vi "Dashboard Main.vi"() -> ()   [LabVIEW 2016]
uses:
  <vilib>/vision/Image Controls.llb/IMAQ Image.ctl
  <vilib>/Utility/miscctls.llb/LVRowAndColumnTypeDef.ctl
  <vilib>/event_ctls.llb/eventvkey.ctl
  <vilib>/Rock Robotics/Network Tables/NT Read Boolean.vi
  <vilib>/Rock Robotics/Network Tables/NT Read Numeric Array.vi
  <vilib>/Rock Robotics/Network Tables/NT Read Boolean Array.vi
  <vilib>/Rock Robotics/WPI/Dashboard/WPI_DashboardLogging Global.vi
  <vilib>/vision/NI_Vision_Development_Module.lvlib
panel:
  in  "Camera Settings Right":T1={"Frame Rate"=30, "Compression"=30, "Size"=1, "DB Camera Config"=FALSE} {"Frame Rate" scale=1.0..30.0; "Compression" scale=100.0..-1.0; "Size" items=["640x480", "320x240", "160x120"]}
  in  "Camera2 Name":string(combo)="Camera2"
  out "Camera Info":cluster{"Mbps LED":bool, "Mbps":dbl, "fps":dbl} {"fps" format="%#.1g"; "Mbps" format="%#.1g"}
  in  "Camera Settings":T1={"Frame Rate"=30, "Compression"=30, "Size"=1, "DB Camera Config"=FALSE} {"Frame Rate" scale=1.0..30.0; "Compression" scale=100.0..-1.0; "Size" items=["640x480", "320x240", "160x120"]}
  in  "TCP":refnum<k5>
  in  "Rec Mode":enum32{"Stop", "Record", "Playback"}(radio)
  out "Robot IP":string
  out "Image Message":string="Timeout in Camera Communications"
  in  "Dashboard Tab":T2(tab)
  in  "Ball Picker Upper Speed":dbl=1.0
  out "Shooter RPM":dbl
  in  "Select Auto":string(combo)="Select Autonomous ..."
  out "NT Connection":bool
  out "MotorChart R":cluster{"Numeric":dbl, "Numeric":dbl}(graph)
  out "MotorChart L":cluster{"Numeric":dbl, "Numeric":dbl}(graph)
  out "MotorSliders R":cluster{"MotorSlide1":dbl, "MotorSlide2":dbl} {"MotorSlide2" scale=-1.0..1.0 scale format="%#_2e"; "MotorSlide1" scale=-1.0..1.0 scale format="%#_2e"}
  out "MotorSliders L":cluster{"MotorSlide1":dbl, "MotorSlide2":dbl} {"MotorSlide2" scale=-1.0..1.0 scale format="%#_2e"; "MotorSlide1" scale=-1.0..1.0 scale format="%#_2e"}
  out "JS1 Z":dbl(slide) scale=-1.0..1.0 scale format="%#_2e"
  out "JS1 Graph":cluster{"X":dbl, "Y":dbl}[](graph)
  out "JS1 Buttons":T3
  out "JS2 Z":dbl(slide) scale=-1.0..1.0 scale format="%#_2e"
  out "JS2 Graph":cluster{"X":dbl, "Y":dbl}[](graph)
  out "JS2 Buttons":T3
  out "Mode":T4(ring)=enum."Auto Disabled"
  out "Drive Direction":enum32{"Gear/Climb", "Ball Picking/Shooting"}(tab)
  out "Gear Holder Position":T5(tab)
  out "Climber Speed":dbl format="%#_2g"
  out "Tab Control":enum32{"Dont Shoot", "SHOOT"}(tab)
  out "Shooter RPM":dbl
  out "Gear Holder Position 2":T6(tab)
  out "LIDAR":dbl
  in  "Drive Forward Auto Wait":dbl
  in  "Distance for 5500RPM":dbl=7.0 format="%#_13g"
  out "Ball Motor Direction":bool
  out "Camera Image Right":T7(plugin-control)
  in  "DB/String 9":string
  in  "DB/String 8":string
  in  "DB/String 7":string
  in  "DB/String 6":string
  in  "DB/String 5":string
  in  "DB/String 4":string
  in  "DB/String 3":string
  in  "DB/String 2":string
  in  "DB/String 1":string
  in  "DB/String 0":string
  in  "DB/Slider 0":dbl(slide) scale=0.0..5.0
  in  "DB/Slider 1":dbl(slide) scale=0.0..5.0
  in  "DB/Slider 2":dbl(slide) scale=0.0..5.0
  in  "DB/Slider 3":dbl(slide) scale=0.0..5.0
  out "DB/LED 3":bool
  out "DB/LED 2":bool
  out "DB/LED 1":bool
  out "DB/LED 0":bool
  in  "DB/Button 3":bool
  in  "DB/Button 2":bool
  in  "DB/Button 1":bool
  in  "DB/Button 0":bool caption="New Name"
  out "Teleop Variables":string[][](array[string])
  in  "Test Slider":dbl(slide) scale=0.0..100.0 scale format="%#_3g"
  in  "On/Off":bool caption="Solenoid"
  in  "Test Name":u16(ring) items=["Select the test to run..."]
  in  "Test Tree":string(tree)
  in  "Motor":cluster{"Value":dbl, "Enable":bool} {"Value" scale=-1.0..1.0 scale format="%#_3g"}
  out "Progress":T8 {"Test Progress" scale=0.0..100.0}
  in  "Rev/Fwd":cluster{"Forward":bool, "Reverse":bool}
  in  "Test Ring":u16(ring) items=["Monochrome", "Color"]
  out "Cmd Status":string
  in  "Execute Command":bool
  in  "Command Params":string[][](table)
  in  "Command Selection":i32(listbox)
  in  "CheckList":i32(listbox)
  out "Tree":string(tree)
  out "Camera Image":T7(plugin-control)
  out "Background":bool
  in  "Camera Name":string(combo)="Camera"
  # "HW"
  # "HW"
  # "Joysticks"
  # "Drive Motors"
  # "Front"
  # "Right"
  # "Left"
  # "Back"
  # "Gear and Climber"
  # "NEITHER SWITCH PRESSED"
  # "Ball Picking/Shooting"
  # "DONT SHOOT"
  # "SHOOT"
  # "This tab is a great place for autonomous settings and robot-specific values.\nPlace controls and indicators inside this tab and match name to\nDashboard Variables on robot. You can also delete this comment."
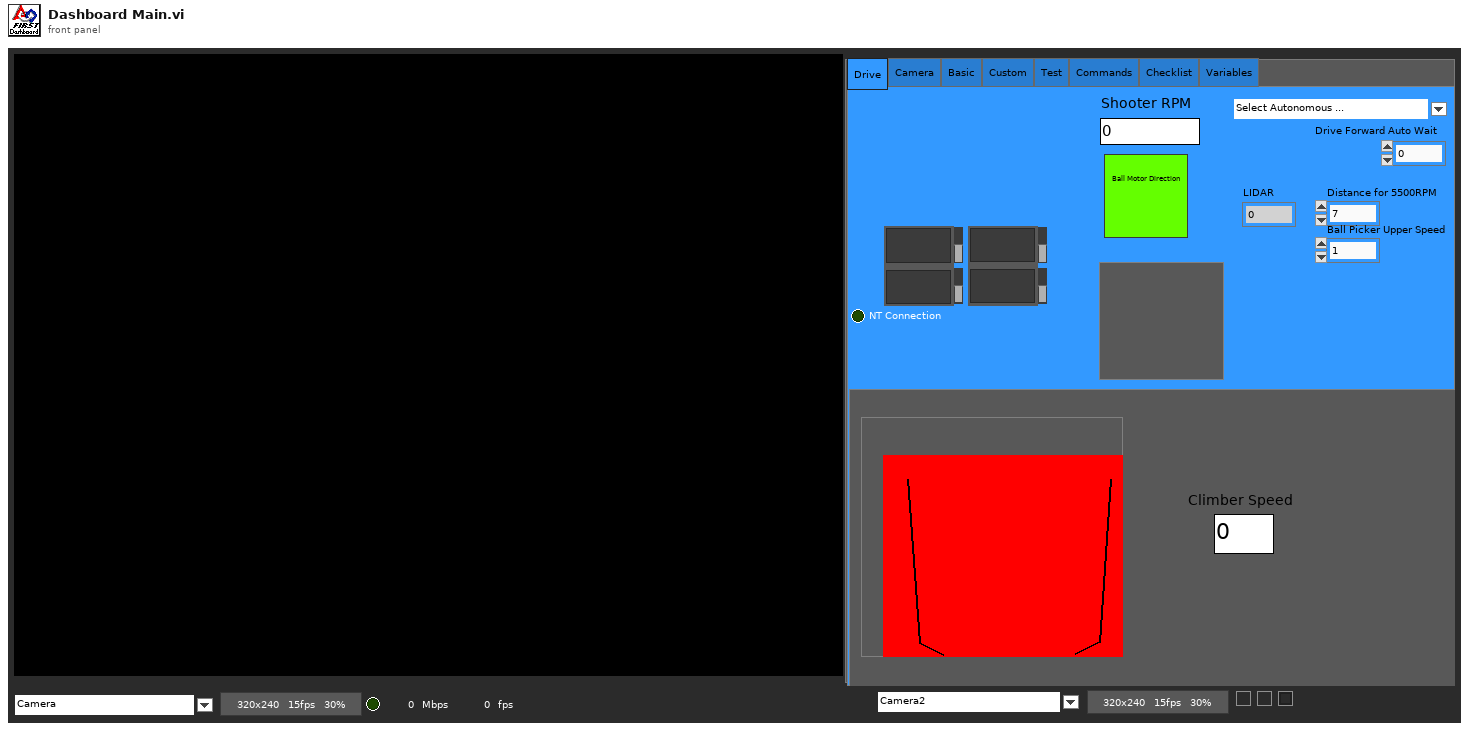
[diagram p1: front panel]
types:
  T1 = cluster{"Frame Rate":i32, "Compression":i32, "Size":u16, "DB Camera Config":bool}
  T2 = enum32{"Drive", "Camera", "Basic", "Custom", "Test", "Commands", "Checklist", "Variables"}
  T3 = cluster{bool, bool, bool, bool, bool, bool, bool, bool, bool, bool, bool, bool}
  T4 = enum8{"Tele-Op Disabled", "Tele-Op Enabled", "Auto Disabled", "Auto Enabled", "Test Disabled", "Test Enabled", "Disconnected", "No Code", "E-Stop"}
  T5 = enum32{"Gear Release Position", "Gear Hold Position", "NA"}
  T6 = enum32{"Gear Release Position", "Gear Hold Position"}
  T7 = typedef "IMAQ Image.ctl" = refnum<image>
  T8 = cluster{"Test Progress":u8, "Test Progress Text":string}
  T9 = typedef "Image Type" = u32
  T10 = cluster{"IDs":cluster{"RPC field ID":u16, "Unique ID":u16}, "String":string}
  T11 = enum32{"Drive", "Basic", "Custom", "Test", "Checklist", "Variables"}
  T12 = cluster{"Camera Image":refnum<vi>, "Dashboard Tab":refnum<vi>, "Background":refnum<vi>, "Rec Mode":refnum<vi>, "Test Slider":refnum<vi>, "On/Off ":refnum<vi>, "Test Ring":refnum<vi>, "Rev/Fwd":refnum<vi>, "Test Name":refnum<vi>, "Motor":refnum<vi>, "Progress":refnum<vi>, "CheckList":refnum<vi>, "Tree":refnum<vi>, "Test Tree":refnum<vi>, "Command Params":refnum<vi>, "Command Selection":refnum<vi>, "Execute Command":refnum<vi>, "Cmd Status":refnum<vi>, "Camera Settings":refnum<vi>, "Camera Name":refnum<vi>, "Camera Info":refnum<vi>, "Camera Settings Right":refnum<vi>, "Camera2 Name":refnum<vi>, "Camera Image Right":refnum<vi>}
  T13 = cluster{"Error Strings":string, "Disable Counts":cluster{u16, u16}, "Rail Faults":cluster{u16, u16, u16}, "Robot IP":string, "DB Mode":u8, "Event Info":cluster{"Name":string, "Type":u8, "Number":u16, "Replay":u8}}
  T14 = cluster{"Storage":cluster{"Disk Free":u64, "RAM Block":u32, "RAM free":u32}, "CPU Utilization":cluster{"CPU % ISR":sgl, "CPU % Time Crit":sgl, "CPU % Timed Str":sgl, "CPU % High":sgl, "CPU % Above":sgl, "CPU % Normal":sgl, "CPU % Low":sgl}, "CAN":cluster{"% Bus Utilization":sgl, "Bus Off Cnt":u32, "TX_FIFO Full Cnt":u32, "Receive Error Cnt":u8, "Transmit Error Cnt":u8}, "HID":cluster{"HID Outputs":u32, "Rumble Low":u16, "Rumble High":u16}[]}
  T15 = cluster{"Status bits":cluster{"Test Mode":bool, "Autonomous":bool, "Enabled":bool, "Code Start":bool, "Brownout":bool, "Reserved 2":bool, "Reserved 3":bool, "E-Stop":bool}, "Code Trace":cluster{"Disabled":bool, "TeleOp":bool, "Auto":bool, "Test":bool}, "Controller Type":enum16{"unknown", "cRIO", "roboRio"}, "Code?":enum16{"unknown", "noCode", "code"}, "Battery V":dbl}
  T16 = cluster{"Control Bits":cluster{"TestMode":bool, "Autonomous":bool, "Enabled":bool, "FMS Present":bool, bool, bool, bool, "E-Stop":bool}, "Team Station ":u8, "Countdown":sgl, "Joystick Values":cluster{"Axes":dbl[], "Buttons":bool[], "POVs":i16[]}[]}
  T17 = cluster{"Axes":dbl[], "Buttons":bool[], "POVs":i16[]}[]
  T18 = cluster{"Axes":dbl[], "Buttons":bool[], "POVs":i16[]}
  T19 = cluster{"Buttons[0]":bool, "Buttons[1]":bool, "Buttons[2]":bool, "Buttons[3]":bool, "Buttons[4]":bool, "Buttons[5]":bool, "Buttons[6]":bool, "Buttons[7]":bool, "Buttons[8]":bool, "Buttons[9]":bool, "Buttons[10]":bool, "Buttons[11]":bool}
  T20 = cluster{"Operation":enum16{"Update", "Clear"}, "Color Box":u32}[]
  T21 = typedef "eventvkey.ctl" = enum16{"ASCII", "Enter", "Return", "Shift", "Ctrl", "Alt", "Cmd", "Opt", "Caps", "NumLock", "Clear", "Break", "Up", "Down", "Left", "Right", "Insert", "Delete", "Home", "End", "PageUp", "PageDown", "Escape", "Help", "Pause", "ScrollLock", "F1", "F2", "F3", "F4", "F5", "F6", "F7", "F8", "F9", "F10", "F11", "F12", "F13", "F14", "F15", "F16", "F17", "F18", "F19", "F20", "F21", "F22", "F23", "F24", "Play", "VolumeUp", "VolumeDown", "Mute", "Two Byte Char"}
  T22 = cluster{"Image Size":bool, "Image Type":bool, "Pixel Value":bool, "ROI Information":bool, "Zoom Factor":bool}
  T23 = cluster{"Operation":enum16{"Update", "Clear"}, "Color Box":u32}
  T24 = typedef "LVRowAndColumnTypeDef.ctl" = cluster{"Row":i32, "Column":i32}
  T25 = cluster{"Shift":bool, "Ctrl":bool, "Alt":bool, "Cmd":bool, "Opt":bool}
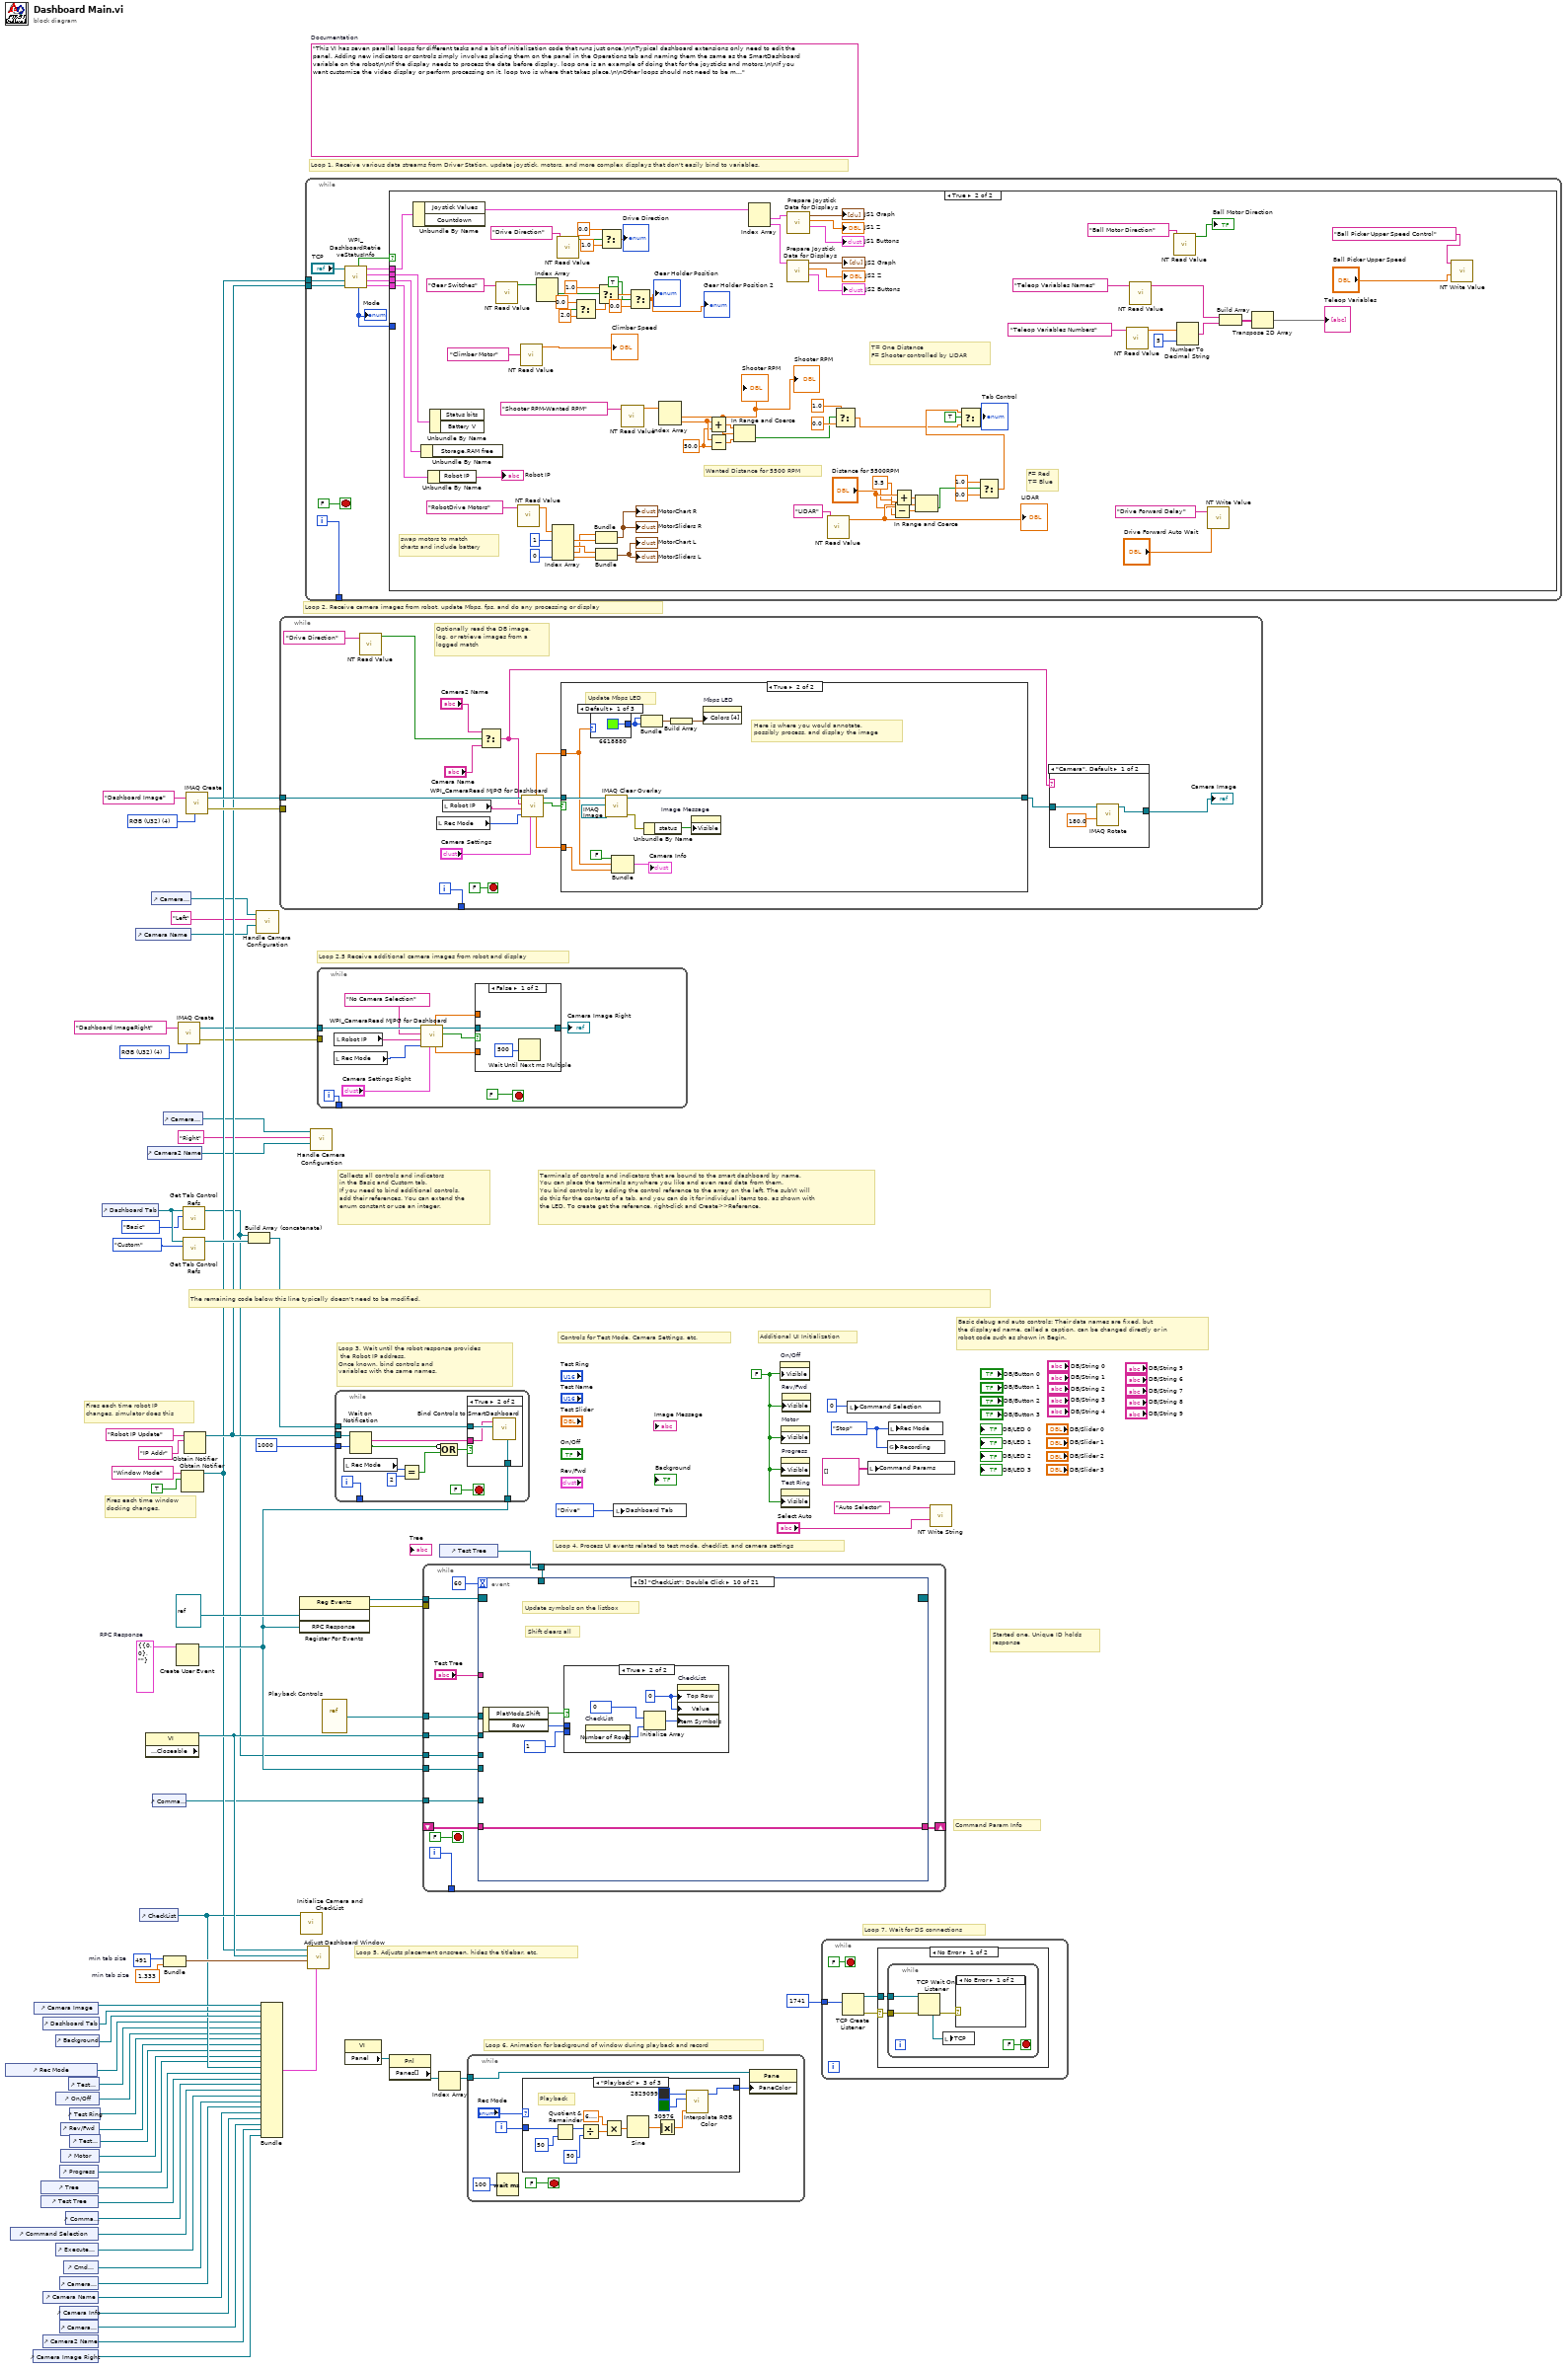
[diagram p0: block diagram]
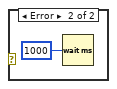
[diagram p3: hidden frame]
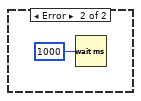
[diagram p4: hidden frame]
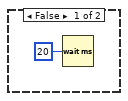
[diagram p5: hidden frame]
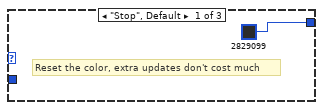
[diagram p6: hidden frame]
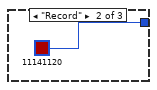
[diagram p7: hidden frame]
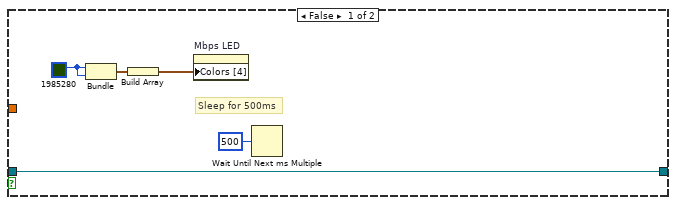
[diagram p10: hidden frame]
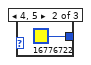
[diagram p11: hidden frame]
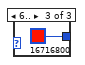
[diagram p12: hidden frame]
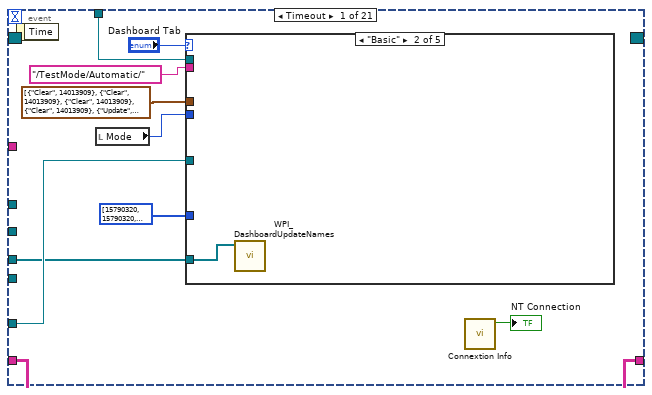
[diagram p13: hidden frame]
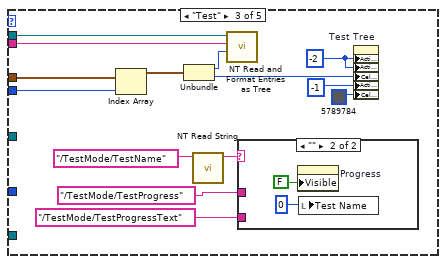
[diagram p15: hidden frame]
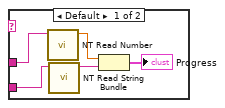
[diagram p16: hidden frame]
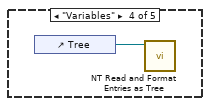
[diagram p17: hidden frame]
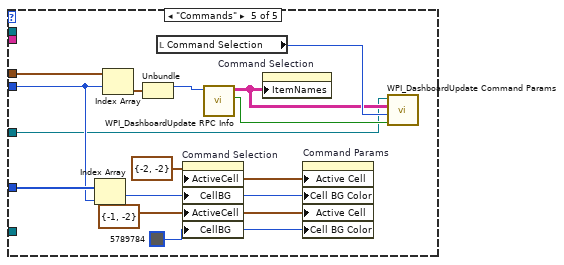
[diagram p18: hidden frame]
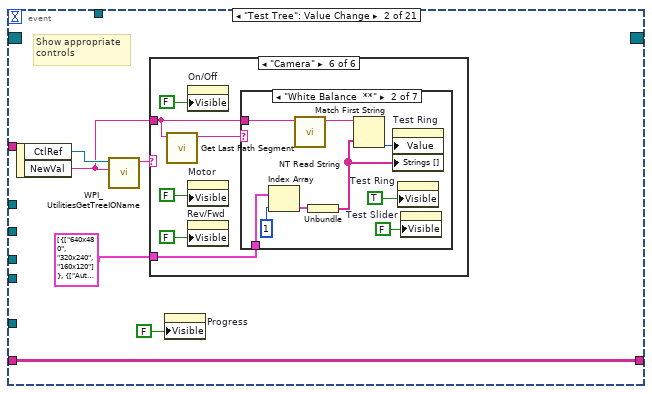
[diagram p19: hidden frame]
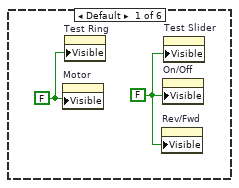
[diagram p20: hidden frame]
diagram:
  (unwired) T7 refnum ("Camera Image")
  w10 = T9 4 items=["Grayscale (U8)", "Grayscale (I16)", "Grayscale (SGL)", "Complex (CSG)", "RGB (U32)", "HSL (U32)", "RGB (U64)"] ("Image Type")
  w26 = T10 {"IDs"={"RPC field ID"=0, "Unique ID"=0}, "String"=""}  # RPC Response
  w51 = 491  # min tab size
  w50 = 1.333  # min tab size
  w58 = enum32{"Stop", "Record", "Playback"}."Stop" ("Rec Mode")
  w33 = FALSE ("Visible")
  (unwired) "This VI has seven parallel loops for different tasks and a bit of initialization code that runs just once.\n\nTypical dashboard extensions only need to edit the panel. Adding new indicators or controls simply involves placing them on the panel in the Operations tab and naming them the same as the SmartDashboard variable on the robot\n\nIf the display needs to process the data before display, loop one is an example of doing that for the joysticks and motors.\n\nIf you want customize the video display or perform processing on it, loop two is where that takes place.\n\nOther loops should not need to be modified. They are pretty standard, and document the task they perform."  # Documentation
  w75 = T9 4 items=["Grayscale (U8)", "Grayscale (I16)", "Grayscale (SGL)", "Complex (CSG)", "RGB (U32)", "HSL (U32)", "RGB (U64)"] ("Image Type")
  # "Loop 2.5 Receive additional camera images from robot and display"
  # "Command Param Info"
  # "Started one, Unique ID holds\nresponse"
  # "Loop 7. Wait for DS connections"
  # "Basic debug and auto controls: Their data names are fixed, but\nthe displayed name, called a caption, can be changed directly or in\nrobot code such as shown in Begin."
  # "Controls for Test Mode, Camera Settings, etc."
  # "Additional UI Initialization"
  # "Loop 6. Animation for background of window during playback and record"
  # "Fires each time robot IP\nchanges, simulator does this"
  # "Fires each time window\ndocking changes."
  # "Collects all controls and indicators\nin the Basic and Custom tab.\nIf you need to bind additional controls,\nadd their references. You can extend the\nenum constant or use an integer."
  # "The remaining code below this line typically doesn't need to be modified."
  # "Loop 4. Process UI events related to test mode, checklist, and camera settings"
  # "Terminals of controls and indicators that are bound to the smart dashboard by name.\nYou can place the terminals anywhere you like and even read data from them.\nYou bind controls by adding the control reference to the array on the left. The subVI will\ndo this for the contents of a tab, and you can do it for individual items too, as shown with\nthe LED. To create get the reference, right-click and Create>>Reference."
  # "Loop 3. Wait until the robot response provides\n the Robot IP address.\nOnce known, bind controls and\nvariables with the same names."
  # "Loop 5. Adjusts placement onscreen, hides the titlebar, etc."
  # "Loop 1. Receive various data streams from Driver Station, update joystick, motors, and more complex displays that don't easily bind to variables."
  # "Loop 2. Receive camera images from robot, update Mbps, fps, and do any processing or display"
  n1 = control-ref of="Rec Mode"() -> (w39:refnum<vi>)
  n2 = control-ref of="Command Selection"() -> (w25:refnum<vi>)
  n3 = control-ref of="Camera Image Right"() -> (w1:refnum<vi>)
  n4 = control-ref of="Camera Image"() -> (w53:refnum<vi>)
  n5 = control-ref of="Tree"() -> (w43:refnum<vi>)
  n6 = control-ref of="Test Tree"() -> (w42:refnum<vi>)
  n7 = control-ref of="Dashboard Tab"() -> (w52:refnum<vi>)
  n8 = control-ref of="Camera Name"() -> (w16:refnum<vi>)
  n9 = control-ref of="Camera2 Name"() -> (w2:refnum<vi>)
  n10 = control-ref of="Execute Command"() -> (w27:refnum<vi>)
  n11 = control-ref of="Background"() -> (w48:refnum<vi>)
  n12 = control-ref of="On/Off"() -> (w37:refnum<vi>)
  n13 = control-ref of="Progress"() -> (w34:refnum<vi>)
  n14 = control-ref of="Camera Settings"() -> (w17:refnum<vi>)
  n15 = control-ref of="Camera Info"() -> (w15:refnum<vi>)
  n16 = control-ref of="Camera Settings Right"() -> (w3:refnum<vi>)
  n17 = control-ref of="Rev/Fwd"() -> (w35:refnum<vi>)
  n18 = control-ref of="Motor"() -> (w40:refnum<vi>)
  n19 = control-ref of="Cmd Status"() -> (w21:refnum<vi>)
  n20 = control-ref of="Command Params"() -> (w28:refnum<vi>)
  n21 = control-ref of="Test Slider"() -> (w38:refnum<vi>)
  n22 = control-ref of="Test Ring"() -> (w36:refnum<vi>)
  n23 = control-ref of="Test Name"() -> (w41:refnum<vi>)
  n24 = control-ref of="Dashboard Tab"() -> (w56:refnum<vi>)
  n25 = control-ref of="Camera Name"() -> (w18:refnum<vi>)
  n26 = control-ref of="CheckList"() -> (w44:refnum<vi>)
  n27 = property class="VI" props=["Front Panel.Closeable"]() -> (reference out=w57:refnum<vi>)  [unwired: 2 in, 2 out]
  n28 = control-ref of="Camera2 Name"() -> (w6:refnum<vi>)
  n29 = control-ref of="Camera Settings"() -> (w19:refnum<vi>)
  n30 = control-ref of="Command Params"() -> (w20:refnum<vi>)
  n31 = control-ref of="Camera Settings Right"() -> (w7:refnum<vi>)
  n32 = Bundle("min tab size"=w51, "min tab size"=w50) -> (w49:cluster{"min tab size":i32, "min tab size":dbl})  [unwired: 1 in]
  n33 = Create User Event(user event datatype=w26) -> (user event=w22:refnum<user-event>)  [unwired: 1 in, 1 out]
  n34 = call "IMAQ Create"("Image Name"="Dashboard ImageRight", "Image Type"=w10) -> ("New Image"=w9:T7, "error out"=w8:errorcluster)  [unwired: 2 in, 1 out]
  n35 = Obtain Notifier(name (unnamed)="Window Mode", notification data type=TRUE) -> (notifier out=w31:refnum<notifier>)  [unwired: 2 in, 2 out]
  n36 = call <vilib>:"Get Tab Control Refs.vi"("Page Index"=T11."Basic" ("Dashboard Tab"), "TabControl in"=w56) -> ("ControlsOnPage"=w14:refnum<vi>[])  [unwired: 9 in]
  n37 = call <vilib>:"Get Tab Control Refs.vi"("Page Index"=T11."Custom" ("Dashboard Tab"), "TabControl in"=w56) -> ("ControlsOnPage"=w55:refnum<vi>[])  [unwired: 9 in]
  n38 = Obtain Notifier(name (unnamed)="Robot IP Update", notification data type="IP Addr" ("name (unnamed)")) -> (notifier out=w32:refnum<notifier>)  [unwired: 2 in, 2 out]
  n39 = call "IMAQ Create"("Image Name"="Dashboard Image", "Image Type"=w75) -> ("New Image"=w73:T7, "error out"=w72:errorcluster)  [unwired: 2 in, 1 out]
  n40 = Build Array (concatenate)(w14, w55) -> (w54:refnum<vi>[])
  n41 = call "Handle Camera Configuration.vi"("CameraNameRef"=w18, "Camera File Name"="Left", "ClusterRef"=w19) -> ()  [unwired: 9 in]
  n42 = Bundle("Camera Image"=w53, "Dashboard Tab"=w52, "Background"=w48, "Rec Mode"=w39, "Test Slider"=w38, "On/Off"=w37, "Test Ring"=w36, "Rev/Fwd"=w35, "Test Name"=w41, "Motor"=w40, "Progress"=w34, "CheckList"=w44, "Tree"=w43, "Test Tree"=w42, "Command Params"=w28, "Command Selection"=w25, "Execute Command"=w27, "Cmd Status"=w21, "Camera Settings"=w17, "Camera Name"=w16, "Camera Info"=w15, "Camera Settings Right"=w3, "Camera2 Name"=w2, "Camera Image Right"=w1) -> (w45:T12)  [unwired: 1 in]
  n43 = while {
    tunnel: w73 -> [w90]
    tunnel: w72 -> [_]
    tunnel: [w91] -> _
    i -> [w91]
    stop <- FALSE stop-if-true
    # "Optionally read the DB image,\nlog, or retrieve images from a\nlogged match"
    n44 = call-poly <vilib>:"NT Read Value.vi"("Name"="Drive Direction") -> ("Boolean"=w77:bool)  [unwired: 9 in, 1 out]
    n45 = local read "Rec Mode"() -> (w86:enum32{"Stop", "Record", "Playback"})
    n46 = local read "Robot IP"() -> (w85:string)
    n47 = Select(t="Camera2 Name", s=w77, f="Camera Name") -> (s? t:f=w76:string)
    n48 = call <vilib>:"WPI_CameraRead MJPG for Dashboard.vi"("Camera Settings"="Camera Settings", "Rec Mode"=w86, "Robot IP"=w85, "Camera Name"=w76, "Refnum in"=w90) -> ("Active"=w88:bool, "Refnum out"=w89:T7, "FPS"=w87:dbl, "Bandwidth (Mbps)"=w84:dbl)  [unwired: 3 in]
    n49 = case shown="True" w88 {
      tunnel: w89 -> [w97 w108]
      tunnel: w84 -> [_ w105]
      tunnel: w87 -> [_ w106]
      tunnel: [w97 w102] -> w78
      frame False {
        w99 = u32 1985280 ("Color Box")
        # "Sleep for 500ms"
        n50 = Bundle("Color Box"=w99, "Color Box"=w99) -> (w100:cluster{"Color Box":u32, "Color Box":u32})  [unwired: 1 out]
        n51 = Build Array(w100) -> (w98:cluster{"Color Box":u32, "Color Box":u32}[])
        n52 = property on="Mbps LED" class="Bool (strict)"("Colors [4]"=w98) -> ()  [unwired: 2 in, 2 out]
        n53 = Wait Until Next ms Multiple(millisecond multiple=u32 500) -> ()  [unwired: 1 out]
      }
      frame True {
        # "Here is where you would annotate,\npossibly process, and display the image"
        # "Update Mbps LED"
        n54 = case shown="Default" w105 {
          tunnel: [u32 6618880 ("Color Box") u32 16776722 ("Color Box") u32 16716800 ("Color Box")] -> w109
          frame Default {
          }
          frame 4, 5 {
          }
          frame 6.. {
          }
        }
        n55 = call "IMAQ Clear Overlay"("Image"=w108) -> ("error out"=w111:errorcluster, "Image Out"=w102:T7)  [unwired: 2 in, 7 out]
        n56 = Bundle(FALSE, "Bandwidth (Mbps)"=w105, "FPS"=w106) -> (→"Camera Info":cluster{bool, "Bandwidth (Mbps)":dbl, "FPS":dbl})  [unwired: 1 in]
        n57 = Bundle("Color Box"=w109, "Color Box"=w109) -> (w110:cluster{"Color Box":u32, "Color Box":u32})  [unwired: 1 out]
        n58 = Unbundle By Name(w111) -> ("status"=w112:bool)
        n59 = Build Array(w110) -> (w107:cluster{"Color Box":u32, "Color Box":u32}[])
        n60 = property on="Image Message" class="Str"("Visible"=w112) -> ()  [unwired: 2 in, 2 out]
        n61 = property on="Mbps LED" class="Bool (strict)"("Colors [4]"=w107) -> ()  [unwired: 2 in, 2 out]
      }
    }
    n62 = case shown="\"Camera\", Default" w76 {
      tunnel: [w94 w96] -> w79
      tunnel: w78 -> [w95 w96]
      frame "Camera", Default {
        n63 = call "IMAQ Rotate"("Angle (degrees)"=sgl 180.0, "Image Src"=w95) -> ("Image Dst Out"=w94:T7)  [unwired: 8 in, 1 out]
      }
      frame "Camera2" {
      }
    }
    "Camera Image" <- w79
  }
  n64 = register-events(refnum<vi> refnum, w22) -> (reference out=w62:refnum<event-registration>, error out=w61:errorcluster)  [unwired: 2 in]
  n65 = call "Initialize Camera and CheckList.vi"("ListBox in"=w44) -> ()  [unwired: 11 in]
  n66 = while {
    tunnel: [w125] -> _
    tunnel: w32 -> [w119]
    tunnel: w31 -> [w116]
    i -> [w125]
    stop <- FALSE stop-if-true
    n67 = call <vilib>:"WPI_DashboardRetrieveStatusInfo.vi"("Binding Refnum"=w119, "Window Mode Notifier"=w116, "TCP Cnx"="TCP") -> ("Power and Errors"=w120:T13, "Robot Metrics"=w123:T14, "Status Info"=w124:T15, "Control Info"=w121:T16, "Robot Mode"=w118:T4, "Process?"=w122:bool)  [unwired: 3 in]
    "Mode" <- w118
    n68 = case shown="True" w122 {
      tunnel: w124 -> [_ w207]
      tunnel: w123 -> [_ w206]
      tunnel: w121 -> [_ w205]
      tunnel: w120 -> [_ w204]
      tunnel: w118 -> [_ _]
      frame False {
        n69 = Wait (ms)(milliseconds to wait=u32 20) -> ()  [unwired: 1 out]
      }
      frame True {
        w133 = 3.5 ("y")
        w149 = 50.0 ("y")
        # "T= One Distance\nF= Shooter controlled by LIDAR"
        # "Wanted Distance for 5500 RPM"
        # "F= Red\nT= Blue"
        # "swap motors to match\ncharts and include battery"
        n70 = Unbundle By Name(w205) -> ("Joystick Values"=w195:T17)  [unwired: 1 out]
        n71 = Unbundle By Name(w206) -> ()  [unwired: 1 out]
        n72 = Unbundle By Name(w204) -> ("Robot IP"=→"Robot IP":string)
        n73 = Unbundle By Name(w207) -> ()  [unwired: 2 out]
        n74 = call-poly <vilib>:"NT Read Value.vi"("Name"="Gear Switches") -> ("Boolean Array"=w167:bool[])  [unwired: 9 in, 1 out]
        n75 = call-poly <vilib>:"NT Read Value.vi"("Name"="RobotDrive Motors") -> ("Numeric Array"=w185:dbl[])  [unwired: 9 in, 1 out]
        n76 = call-poly <vilib>:"NT Read Value.vi"("Name"="Climber Motor") -> ("Numeric"=→"Climber Speed":dbl)  [unwired: 9 in, 1 out]
        n77 = Index Array(array=w167) -> (element #1=w166:bool, element #2=w164:bool)  [unwired: 2 in]
        n78 = Index Array(array=w185, index #1=1, index #4=0) -> (element #1=w199:dbl, element #2=w200:dbl, element #3=w198:dbl, element #4=w203:dbl)  [unwired: 2 in]
        n79 = call-poly <vilib>:"NT Read Value.vi"("Name"="Drive Direction") -> ("Boolean"=w172:bool)  [unwired: 9 in, 1 out]
        n80 = Select(t=0.0, s=w164, f=2.0) -> (s? t:f=w163:dbl)
        n81 = Bundle("Numeric"=w198, "Numeric"=w199) -> (→"MotorChart R" →"MotorSliders R":cluster{"Numeric":dbl, "Numeric":dbl})  [unwired: 1 in]
        n82 = Bundle("Numeric"=w200, "Numeric"=w203) -> (→"MotorChart L" →"MotorSliders L":cluster{"Numeric":dbl, "Numeric":dbl})  [unwired: 1 in]
        n83 = Select(t=1.0, s=w166, f=w163) -> (s? t:f=w158:dbl)
        n84 = Select(t=0.0, s=w172, f=1.0) -> (s? t:f=→"Drive Direction":dbl)
        n85 = call-poly <vilib>:"NT Read Value.vi"("Name"="Shooter RPM-Wanted RPM") -> ("Numeric Array"=w155:dbl[])  [unwired: 9 in, 1 out]
        n86 = Select(t=w158, s=TRUE, f=0.0) -> (s? t:f=→"Gear Holder Position" →"Gear Holder Position 2":dbl)
        n87 = Index Array(array=w155) -> (element #1=w147:dbl, element #2=w150:dbl)  [unwired: 2 in]
        "Shooter RPM" <- w147
        "Shooter RPM" <- w147
        n88 = Add(x=w150, y=w149) -> (x+y=w152:dbl)
        n89 = Subtract(x=w150, y=w149) -> (x-y=w151:dbl)
        n90 = In Range and Coerce(upper limit=w152, x=w147, lower limit=w151) -> (In Range?=w148:bool)  [unwired: 1 out]
        n91 = Index Array(array=w195) -> (element #1=w194:T18, element #2=w190:T18)  [unwired: 2 in]
        n92 = call "Prepare Joystick Data for Displays.vi"("Joystick Values"=w190) -> ("Buttons"=→"JS2 Buttons":T19, "Z Axis"=→"JS2 Z":dbl, "Cartesian Data"=→"JS2 Graph":cluster{"X axis":dbl, "X axis":dbl}[])  [unwired: 8 in]
        n93 = call "Prepare Joystick Data for Displays.vi"("Joystick Values"=w194) -> ("Buttons"=→"JS1 Buttons":T19, "Z Axis"=→"JS1 Z":dbl, "Cartesian Data"=→"JS1 Graph":cluster{"X axis":dbl, "X axis":dbl}[])  [unwired: 8 in]
        n94 = call-poly <vilib>:"NT Read Value.vi"("Name"="LIDAR") -> ("Numeric"=w137:dbl)  [unwired: 9 in, 1 out]
        "LIDAR" <- w137
        n95 = Select(t=1.0, s=w148, f=0.0) -> (s? t:f=w128:dbl)
        n96 = Subtract(x="Distance for 5500RPM", y=w133) -> (x-y=w135:dbl)
        n97 = Add(x="Distance for 5500RPM", y=w133) -> (x+y=w136:dbl)
        n98 = In Range and Coerce(upper limit=w136, x=w137, lower limit=w135) -> (In Range?=w132:bool)  [unwired: 1 out]
        n99 = Select(t=1.0, s=w132, f=0.0) -> (s? t:f=w129:dbl)
        n100 = Select(t=w129, s=TRUE, f=w128) -> (s? t:f=→"Tab Control":dbl)
        n101 = call-poly <vilib>:"NT Read Value.vi"("Name"="Teleop Variables Numbers") -> ("Numeric Array"=w178:dbl[])  [unwired: 9 in, 1 out]
        n102 = call-poly <vilib>:"NT Read Value.vi"("Name"="Teleop Variables Names") -> ("String Array"=w179:string[])  [unwired: 9 in, 1 out]
        n103 = call-poly <vilib>:"NT Read Value.vi"("Name"="Ball Motor Direction") -> ("Boolean"=→"Ball Motor Direction":bool)  [unwired: 9 in, 1 out]
        n104 = Number To Decimal String(number=w178, width (-)=i16 5) -> (decimal integer string=w176:string[])
        n105 = call-poly <vilib>:"NT Write Value.vi"("Numeric"="Drive Forward Auto Wait", "Name"="Drive Forward Delay") -> ()  [unwired: 9 in, 1 out]
        n106 = Build Array(w179, w176) -> (w175:string[][])
        n107 = Transpose 2D Array(2D array=w175) -> (transposed array=→"Teleop Variables":string[][])
        n108 = call-poly <vilib>:"NT Write Value.vi"("Numeric"="Ball Picker Upper Speed", "Name"="Ball Picker Upper Speed Control") -> ()  [unwired: 9 in, 1 out]
      }
    }
  }
  n109 = call "Adjust Dashboard Window.vi"("Sizing Refnums"=w45, "Size Constraints"=w49, "VI"=w57, "WIn Mode"=w31) -> ()  [unwired: 8 in]
  n110 = call "Handle Camera Configuration.vi"("CameraNameRef"=w6, "Camera File Name"="Right", "ClusterRef"=w7) -> ()  [unwired: 9 in]
  n111 = while {
    tunnel: w9 -> [w219]
    tunnel: w8 -> [_]
    tunnel: [w213] -> _
    i -> [w213]
    stop <- FALSE stop-if-true
    n112 = local read "Rec Mode"() -> (w217:enum32{"Stop", "Record", "Playback"})
    n113 = local read "Robot IP"() -> (w218:string)
    n114 = call <vilib>:"WPI_CameraRead MJPG for Dashboard.vi"("Camera Settings"="Camera Settings Right", "Rec Mode"=w217, "Robot IP"=w218, "Camera Name"="No Camera Selection", "Refnum in"=w219) -> ("Active"=w212:bool, "Refnum out"=w215:T7, "FPS"=w210:dbl, "Bandwidth (Mbps)"=w211:dbl)  [unwired: 3 in]
    n115 = case shown="False" w212 {
      tunnel: w215 -> [w220 w222]
      tunnel: w211 -> [_ _]
      tunnel: w210 -> [_ _]
      tunnel: [w220 w222] -> w209
      frame False {
        n116 = Wait Until Next ms Multiple(millisecond multiple=u32 500) -> ()  [unwired: 1 out]
      }
      frame True {
      }
    }
    "Camera Image Right" <- w209
  }
  n117 = vi-ref "Playback Controls.vi"() -> (w63:refnum<vi>)
  n118 = while {
    tunnel: w54 -> [w234]
    tunnel: w32 -> [w232]
    tunnel: [w230] -> _
    tunnel: u32 1000 ("milliseconds to wait") -> [w229]
    tunnel: w22 -> [w223]
    i -> [w230]
    stop <- FALSE stop-if-true
    n119 = local read "Rec Mode"() -> (w225:enum32{"Stop", "Record", "Playback"})
    n120 = Wait on Notification(notifier=w232, timeout in ms (-1)=w229) -> (notification=w231:string, timed out?=w227:bool)  [unwired: 2 in, 2 out]
    n121 = Equal?(x=w225, y=u16 2 ("Rec Mode")) -> (x = y?=w226:bool)
    n122 = Compound Arithmetic op=OR(invert w227, w226) -> (w228:bool)
    n123 = case shown="True" w228 {
      tunnel: w234 -> [_ w237]
      tunnel: w231 -> [_ w236]
      tunnel: w223 -> [_ w235]
      frame False {
      }
      frame True {
        n124 = call <vilib>:"Bind Controls to SmartDashboard.vi"("RPC ref"=w235, "Bound Control Refs"=w237, "Server IP Address"=w236) -> ()  [unwired: 9 in]
      }
    }
  }
  n125 = property class="VI"() -> ("Panel"=w65:refnum<vi>)  [unwired: 2 in, 2 out]
  n126 = property class="Pnl"(reference=w65) -> ("Panes[]"=w66:refnum<vi>[])  [unwired: 1 in, 2 out]
  n127 = Index Array(array=w66) -> (element=w64:refnum<vi>)  [unwired: 1 in]
  n128 = control-ref of="Test Tree"() -> (w67:refnum<vi>)
  n129 = while {
    tunnel: [w247] -> _
    tunnel: w67 -> [w246]
    tunnel: w63 -> [w245]
    tunnel: w62 -> [w244]
    tunnel: w61 -> [_]
    tunnel: w57 -> [w243]
    tunnel: w22 -> [w242]
    tunnel: w20 -> [w241]
    shift-right: [w240] -> _
    shift-left: _ -> [w239]
    tunnel: w14 -> [w238]
    i -> [w247]
    stop <- FALSE stop-if-true
    n130 = event shown="[9] \"CheckList\": Double Click" {
      selector: w244 -> [_ _ _ _ _ _ _ _ _ _ _ _ _ _ _ _ _ _ _ _ _]
      dyn-events: [_ _ _ _ _ _ _ _ _ _ _ _ _ _ _ _ w503 _ _ _ _] -> _
      timeout: u32 60 ("milliseconds to wait") -> [_ _ _ _ _ _ _ _ _ _ _ _ _ _ _ _ _ _ _ _ _]
      tunnel: w246 -> [w259 _ _ _ _ _ _ _ _ _ _ _ _ _ _ _ _ _ _ _ _]
      tunnel: "Test Tree" -> [_ _ _ _ _ _ _ _ _ _ _ w470 w478 w480 w484 w492 _ _ _ _ _]
      tunnel: w245 -> [_ _ _ _ _ _ _ _ _ _ _ _ _ _ _ _ w505 _ w523 _ _]
      tunnel: w243 -> [_ _ _ _ _ _ _ _ _ _ _ _ _ _ _ _ w501 _ _ _ _]
      tunnel: w242 -> [_ _ _ _ _ _ _ _ _ _ _ _ _ _ _ _ w497 _ _ _ _]
      tunnel: w241 -> [w254 _ _ _ _ _ w421 _ _ _ _ _ _ _ _ _ _ _ _ _ _]
      tunnel: [w253 w298 w400 w405 w414 w418 w419 w428 w438 w445 w457 w469 w476 w479 w483 w491 w496 w518 w520 w524 w535] -> w240
      tunnel: w239 -> [w253 w298 w400 w405 w414 w418 w419 _ _ w445 w457 w469 w476 w479 w483 w491 w496 w518 w520 w524 w535]
      tunnel: w238 -> [w251 _ _ _ _ _ _ _ _ _ _ _ _ _ _ _ _ _ _ _ _]
      event Timeout {
        n131 = event-data() -> ()  [unwired: 1 in, 1 out]
        n132 = local read "Mode"() -> (w256:T4)
        n133 = case shown="\"Basic\"" "Dashboard Tab" {
          tunnel: w259 -> [_ _ w275 _ _]
          tunnel: "/TestMode/Automatic/" ("Name Pattern") -> [_ _ w274 _ _]
          tunnel: T20 [{"Operation"=enum."Clear", "Color Box"=14013909}, {"Operation"=enum."Clear", "Color Box"=14013909}, {"Operation"=enum."Clear", "Color Box"=14013909}, {"Operation"=enum."Clear", "Color Box"=14013909}, {"Operation"=enum."Update", "Color Box"=14013909}, {"Operation"=enum."Update", "Color Box"=16777215}, {"Operation"=enum."Clear", "Color Box"=14013909}, {"Operation"=enum."Clear", "Color Box"=14013909}, {"Operation"=enum."Clear", "Color Box"=14013909}] -> [_ _ w267 _ w291]
          tunnel: w256 -> [_ _ w266 _ w290]
          tunnel: u32[] [15790320, 15790320, 15790320, 15790320, 16777215, 16777215, 15790320, 15790320, 15790320] -> [_ _ _ _ w296]
          tunnel: w254 -> [_ _ _ _ w284]
          tunnel: w251 -> [_ w261 _ _ _]
          frame "Custom", Default {
          }
          frame "Basic" {
            n134 = call <vilib>:"WPI_DashboardUpdateNames.vi"("Controls on Tab"=w261) -> ()  [unwired: 11 in]
          }
          frame "Test" {
            w273 = -2 ("Active Item:Row Number")
            n135 = Index Array(array=w267, index=w266) -> (element=w268:T23)
            n136 = Unbundle(w268) -> ("Operation"=w269:enum16{"Update", "Clear"}, "Color Box"=w270:u32)
            n137 = call <vilib>:"NT Read String.vi"("Name"="/TestMode/TestName") -> ("String"=w264:string)  [unwired: 9 in, 1 out]
            n138 = call <vilib>:"NT Read and Format Entries as Tree.vi"("Operation"=w269, "Name Pattern"=w274, "Tree Refnum"=w275) -> ()  [unwired: 7 in, 2 out]
            n139 = case shown="\"\"" w264 {
              tunnel: "/TestMode/TestProgress" ("Name") -> [w277 _]
              tunnel: "/TestMode/TestProgressText" ("Name") -> [w276 _]
              frame Default {
                n140 = call <vilib>:"NT Read Number.vi"("Name"=w277) -> ("Numeric"=w278:dbl)  [unwired: 9 in, 1 out]
                n141 = call <vilib>:"NT Read String.vi"("Name"=w276) -> ("String"=w279:string)  [unwired: 9 in, 1 out]
                n142 = Bundle("Numeric"=w278, "String"=w279) -> (→"Progress":cluster{"Numeric":dbl, "String":string})  [unwired: 1 in]
              }
              frame "" {
                n143 = property on="Progress" class="Clust (strict)"("Visible"=FALSE) -> ()  [unwired: 2 in, 2 out]
                n144 = local write "Test Name"(u16 0) -> ()
              }
            }
            n145 = property on="Test Tree" class="Tree (strict)"("Active Item Row Number"=w273, "ActiveColNum"=w273, "CellBG"=w270, "Active Item Row Number"=-1 ("Active Item:Row Number"), "CellBG"=u32 5789784 ("Color Box")) -> ()  [unwired: 2 in, 2 out]
          }
          frame "Variables" {
            n146 = control-ref of="Tree"() -> (w283:refnum<vi>)
            n147 = call <vilib>:"NT Read and Format Entries as Tree.vi"("Tree Refnum"=w283) -> ()  [unwired: 9 in, 2 out]
          }
          frame "Commands" {
            w292 = u32 5789784 ("Color Box")
            w293 = T24 {"Row"=-1, "Column"=-2} ("Active Cell:Active Cell")
            w295 = T24 {"Row"=-2, "Column"=-2} ("Active Cell:Active Cell")
            n148 = Index Array(array=w296, index=w290) -> (element=w294:u32)
            n149 = Index Array(array=w291, index=w290) -> (element=w289:T23)
            n150 = Unbundle(w289) -> ("Operation"=w288:enum16{"Update", "Clear"})  [unwired: 1 out]
            n151 = local read "Command Selection"() -> (w287:i32)
            n152 = property on="Command Selection" class="MCListbox (strict)"("ActiveCell"=w295, "CellBG"=w294, "ActiveCell"=w293, "CellBG"=w292) -> ()  [unwired: 2 in, 2 out]
            n153 = call <vilib>:"WPI_DashboardUpdate RPC Info.vi"("Operation"=w288) -> ("update"=w286:bool, "commands"=w285:string[][])  [unwired: 9 in]
            n154 = property on="Command Selection" class="MCListbox (strict)"("ItemNames"=w285) -> ()  [unwired: 2 in, 2 out]
            n155 = property on="Command Params" class="Tbl (strict)"("Active Cell"=w295, "Cell BG Color"=w294, "Active Cell"=w293, "Cell BG Color"=w292) -> ()  [unwired: 2 in, 2 out]
            n156 = call <vilib>:"WPI_DashboardUpdate Command Params.vi"("Update"=w286, "NewVal"=w287, "Commands"=w285, "Param Tbl"=w284) -> ()  [unwired: 7 in, 1 out]
          }
        }
        n157 = call <vilib>:"Connextion Info.vi"() -> ("Connected"=→"NT Connection":bool)  [unwired: 10 in, 1 out]
      }
      event "Test Tree": Value Change {
        # "Show appropriate\ncontrols"
        n158 = event-data() -> ("CtlRef"=w301:refnum<vi>, "NewVal"=w299:string)  [unwired: 1 in]
        n159 = call <vilib>:"WPI_UtilitiesGetTreeIOName.vi"("NewVal"=w299, "TreeControl in"=w301) -> ("I/O Name"=w302:string)  [unwired: 9 in]
        n160 = case shown="\"Camera\"" w302 {
          selector: w302 -> [_ w309 _ w331 w340 _]
          tunnel: w299 -> [_ _ w328 w330 _ w347]
          tunnel: cluster{string[]}[] [{["640x480", "320x240", "160x120"]}, {["Auto", "Fixed indoor", "Fixed outdoor 1", "Fixed outdoor 2", "Fixed fluorescent 1", "Fixed fluorescent 2", "Hold current"]}, {["Auto", "Flicker-free 50 Hz", "Flicker-free 60 Hz", "Hold current"]}, {["None", "Prioritize frame rate", "Prioritize image quality"]}, {["Monochrome", "Color"]}] -> [_ _ _ _ _ w346]
          frame Default {
            w304 = FALSE ("Visible")
            w303 = FALSE ("Visible")
            n161 = property on="Motor" class="Clust (strict)"("Visible"=w303) -> ()  [unwired: 2 in, 2 out]
            n162 = property on="Test Ring" class="Ring (strict)"("Visible"=w303) -> ()  [unwired: 2 in, 2 out]
            n163 = property on="Rev/Fwd" class="Clust (strict)"("Visible"=w304) -> ()  [unwired: 2 in, 2 out]
            n164 = property on="On/Off" class="Bool (strict)"("Visible"=w304) -> ()  [unwired: 2 in, 2 out]
            n165 = property on="Test Slider" class="Slide (strict)"("Visible"=w304) -> ()  [unwired: 2 in, 2 out]
          }
          frame "Analog Out", "Motor", "PWM" {
            w310 = FALSE ("Visible")
            n166 = case shown="\"Analog Out\"" w309 {
              tunnel: [1.0 ("Value") -1.0 ("Value") 0.0 ("Value")] -> w308
              tunnel: [255.0 ("Value") 1.0 ("Value") 5.0 ("Value")] -> w307
              tunnel: [128.0 ("Value") 0.0 ("Value") 0.0 ("Value")] -> w306
              tunnel: [64.0 ("Value") 0.5 ("Value") 1.0 ("Value")] -> w305
              frame "PWM" {
              }
              frame "Motor", Default {
              }
              frame "Analog Out" {
              }
            }
            n167 = property on="Motor" class="Clust (strict)"("Visible"=TRUE) -> ()  [unwired: 2 in, 2 out]
            n168 = property on="Value" class="Slide (strict)"("Value"=w306, "Scale.Minimum"=w308, "Scale.Maximum"=w307, "Scale.Increment"=w305) -> ()  [unwired: 2 in, 2 out]
            n169 = property on="On/Off" class="Bool (strict)"("Visible"=w310) -> ()  [unwired: 2 in, 2 out]
            n170 = property on="Test Slider" class="Slide (strict)"("Visible"=w310) -> ()  [unwired: 2 in, 2 out]
            n171 = property on="Test Ring" class="Ring (strict)"("Visible"=w310) -> ()  [unwired: 2 in, 2 out]
            n172 = property on="Rev/Fwd" class="Clust (strict)"("Visible"=w310) -> ()  [unwired: 2 in, 2 out]
          }
          frame "Servo" {
            w326 = FALSE ("Visible")
            n173 = call <vilib>:"NT Read Number.vi"("Name"=w328) -> ("Numeric"=w327:dbl)  [unwired: 9 in, 1 out]
            n174 = property on="Test Slider" class="Slide (strict)"("Visible"=TRUE, "Scale.Maximum"=170.0 ("Scale.Range:Maximum")) -> ()  [unwired: 2 in, 2 out]
            n175 = local write "Test Slider"(w327) -> ()
            n176 = property on="Motor" class="Clust (strict)"("Visible"=w326) -> ()  [unwired: 2 in, 2 out]
            n177 = property on="Rev/Fwd" class="Clust (strict)"("Visible"=w326) -> ()  [unwired: 2 in, 2 out]
            n178 = property on="On/Off" class="Bool (strict)"("Visible"=w326) -> ()  [unwired: 2 in, 2 out]
            n179 = property on="Test Ring" class="Ring (strict)"("Visible"=w326) -> ()  [unwired: 2 in, 2 out]
          }
          frame "Relay", "Solenoid" {
            w329 = FALSE ("Visible")
            n180 = property on="Motor" class="Clust (strict)"("Visible"=w329) -> ()  [unwired: 2 in, 2 out]
            n181 = property on="Test Slider" class="Slide (strict)"("Visible"=w329) -> ()  [unwired: 2 in, 2 out]
            n182 = Search and Replace String(input string=w330, search string="/Value  **", replace string="/Direction") -> (result string=w336:string)  [unwired: 5 in, 3 out]
            n183 = property on="Test Ring" class="Ring (strict)"("Visible"=w329) -> ()  [unwired: 2 in, 2 out]
            n184 = call <vilib>:"NT Read String.vi"("Name"=w336) -> ("String"=w334:string)  [unwired: 9 in, 1 out]
            n185 = Equal?(x="Both directions", y=w334) -> (x = y?=w332:bool)
            n186 = Not(x=w332) -> (.not. x?=w333:bool)
            n187 = property on="Rev/Fwd" class="Clust (strict)"("Visible"=w332) -> ()  [unwired: 2 in, 2 out]
            n188 = property on="On/Off" class="Bool (strict)"("Visible"=w333, "Caption.Text"=w331) -> ()  [unwired: 2 in, 2 out]
          }
          frame "Compressor", "Digital Out" {
            w339 = FALSE ("Visible")
            # "Get direction and finish"
            n189 = property on="Motor" class="Clust (strict)"("Visible"=w339) -> ()  [unwired: 2 in, 2 out]
            n190 = property on="Test Slider" class="Slide (strict)"("Visible"=w339) -> ()  [unwired: 2 in, 2 out]
            n191 = property on="Test Ring" class="Ring (strict)"("Visible"=w339) -> ()  [unwired: 2 in, 2 out]
            n192 = property on="On/Off" class="Bool (strict)"("Visible"=TRUE, "Caption.Text"=w340) -> ()  [unwired: 2 in, 2 out]
            n193 = property on="Rev/Fwd" class="Clust (strict)"("Visible"=FALSE) -> ()  [unwired: 2 in, 2 out]
          }
          frame "Camera" {
            n194 = call <vilib>:"Get Last Path Segment.vi"("String in"=w347) -> ("String out"=w348:string)  [unwired: 10 in]
            n195 = property on="On/Off" class="Bool (strict)"("Visible"=FALSE) -> ()  [unwired: 2 in, 2 out]
            n196 = property on="Motor" class="Clust (strict)"("Visible"=FALSE) -> ()  [unwired: 2 in, 2 out]
            n197 = property on="Rev/Fwd" class="Clust (strict)"("Visible"=FALSE) -> ()  [unwired: 2 in, 2 out]
            n198 = case shown="\"White Balance  **\"" w348 {
              tunnel: w347 -> [w354 w363 w372 w381 w390 _ w396]
              tunnel: w346 -> [w352 w360 w369 w378 w387 _ _]
              frame "Size  **" {
                n199 = Index Array(array=w352) -> (element=w351:cluster{string[]})  [unwired: 1 in]
                n200 = call <vilib>:"NT Read String.vi"("Name"=w354) -> ("String"=w353:string)  [unwired: 9 in, 1 out]
                n201 = Unbundle(w351) -> (w349:string[])
                n202 = Match First String(2:w349, 3:w353) -> (0:w350:i32)  [unwired: 1 out]
                n203 = property on="Test Ring" class="Ring (strict)"("Value"=w350, "Strings []"=w349) -> ()  [unwired: 2 in, 2 out]
                n204 = property on="Test Ring" class="Ring (strict)"("Visible"=TRUE) -> ()  [unwired: 2 in, 2 out]
                n205 = property on="Test Slider" class="Slide (strict)"("Visible"=FALSE) -> ()  [unwired: 2 in, 2 out]
              }
              frame "White Balance  **" {
                n206 = Index Array(array=w360, index=1) -> (element=w361:cluster{string[]})
                n207 = call <vilib>:"NT Read String.vi"("Name"=w363) -> ("String"=w362:string)  [unwired: 9 in, 1 out]
                n208 = Unbundle(w361) -> (w358:string[])
                n209 = Match First String(2:w358, 3:w362) -> (0:w357:i32)  [unwired: 1 out]
                n210 = property on="Test Ring" class="Ring (strict)"("Value"=w357, "Strings []"=w358) -> ()  [unwired: 2 in, 2 out]
                n211 = property on="Test Ring" class="Ring (strict)"("Visible"=TRUE) -> ()  [unwired: 2 in, 2 out]
                n212 = property on="Test Slider" class="Slide (strict)"("Visible"=FALSE) -> ()  [unwired: 2 in, 2 out]
              }
              frame "Exposure  **" {
                n213 = Index Array(array=w369, index=2) -> (element=w370:cluster{string[]})
                n214 = call <vilib>:"NT Read String.vi"("Name"=w372) -> ("String"=w371:string)  [unwired: 9 in, 1 out]
                n215 = Unbundle(w370) -> (w366:string[])
                n216 = Match First String(2:w366, 3:w371) -> (0:w367:i32)  [unwired: 1 out]
                n217 = property on="Test Ring" class="Ring (strict)"("Value"=w367, "Strings []"=w366) -> ()  [unwired: 2 in, 2 out]
                n218 = property on="Test Ring" class="Ring (strict)"("Visible"=TRUE) -> ()  [unwired: 2 in, 2 out]
                n219 = property on="Test Slider" class="Slide (strict)"("Visible"=FALSE) -> ()  [unwired: 2 in, 2 out]
              }
              frame "Exposure Priority  **" {
                n220 = Index Array(array=w378, index=3) -> (element=w379:cluster{string[]})
                n221 = call <vilib>:"NT Read String.vi"("Name"=w381) -> ("String"=w380:string)  [unwired: 9 in, 1 out]
                n222 = Unbundle(w379) -> (w375:string[])
                n223 = Match First String(2:w375, 3:w380) -> (0:w376:i32)  [unwired: 1 out]
                n224 = property on="Test Ring" class="Ring (strict)"("Value"=w376, "Strings []"=w375) -> ()  [unwired: 2 in, 2 out]
                n225 = property on="Test Ring" class="Ring (strict)"("Visible"=TRUE) -> ()  [unwired: 2 in, 2 out]
                n226 = property on="Test Slider" class="Slide (strict)"("Visible"=FALSE) -> ()  [unwired: 2 in, 2 out]
              }
              frame "Color Enable  **" {
                n227 = Index Array(array=w387, index=4) -> (element=w388:cluster{string[]})
                n228 = call <vilib>:"NT Read String.vi"("Name"=w390) -> ("String"=w389:string)  [unwired: 9 in, 1 out]
                n229 = Unbundle(w388) -> (w384:string[])
                n230 = Match First String(2:w384, 3:w389) -> (0:w385:i32)  [unwired: 1 out]
                n231 = property on="Test Ring" class="Ring (strict)"("Value"=w385, "Strings []"=w384) -> ()  [unwired: 2 in, 2 out]
                n232 = property on="Test Ring" class="Ring (strict)"("Visible"=TRUE) -> ()  [unwired: 2 in, 2 out]
                n233 = property on="Test Slider" class="Slide (strict)"("Visible"=FALSE) -> ()  [unwired: 2 in, 2 out]
              }
              frame Default {
                n234 = property on="Test Ring" class="Ring (strict)"("Visible"=FALSE) -> ()  [unwired: 2 in, 2 out]
                n235 = property on="Test Slider" class="Slide (strict)"("Visible"=FALSE) -> ()  [unwired: 2 in, 2 out]
              }
              frame "Brightness  **", "Color Level  **", "Compression  **", "FPS  **", "Sharpness  **" {
                n236 = call <vilib>:"NT Read Number.vi"("Name"=w396) -> ("Numeric"=w395:dbl)  [unwired: 9 in, 1 out]
                n237 = local write "Test Slider"(w395) -> ()
                n238 = property on="Test Slider" class="Slide (strict)"("Visible"=TRUE, "Scale.Maximum"=100.0 ("Scale.Range:Maximum")) -> ()  [unwired: 2 in, 2 out]
                n239 = property on="Test Ring" class="Ring (strict)"("Visible"=FALSE) -> ()  [unwired: 2 in, 2 out]
              }
            }
          }
        }
        n240 = property on="Progress" class="Clust (strict)"("Visible"=FALSE) -> ()  [unwired: 2 in, 2 out]
      }
      event "Test Name": Mouse Enter {
        # "Populate the ring with the list of tests"
        n241 = event-data() -> ()  [unwired: 1 in, 1 out]
        n242 = call <vilib>:"NT Read String Array.vi"("Name"="/TestMode/TestList") -> ("String Array"=w404:string[])  [unwired: 9 in, 1 out]
        n243 = Build Array (concatenate)("Select the test to run...", w404) -> (w403:string[])
        n244 = property on="Test Name" class="Ring (strict)"("Strings []"=w403) -> ()  [unwired: 2 in, 2 out]
      }
      event "Test Name": Value Change {
        w406 = FALSE ("Visible")
        # "Tell the robot the test name to run"
        n245 = event-data() -> ("NewVal"=w410:u16)  [unwired: 1 in]
        n246 = property on="Test Name" class="Ring (strict)"() -> ("Strings []"=w411:string[])  [unwired: 2 in, 2 out]
        n247 = local write "Progress"(T8 {"Test Progress"=0, "Test Progress Text"=""} ("Progress")) -> ()
        n248 = Index Array(array=w411, index=w410) -> (element=w409:string)
        n249 = call <vilib>:"NT Write String.vi"("String"=w409, "Name"="/TestMode/TestName") -> ()  [unwired: 9 in, 1 out]
        n250 = property on="Progress" class="Clust (strict)"("Visible"=TRUE) -> ()  [unwired: 2 in, 2 out]
        n251 = property on="Motor" class="Clust (strict)"("Visible"=w406) -> ()  [unwired: 2 in, 2 out]
        n252 = property on="Test Slider" class="Slide (strict)"("Visible"=w406) -> ()  [unwired: 2 in, 2 out]
        n253 = property on="On/Off" class="Bool (strict)"("Visible"=w406) -> ()  [unwired: 2 in, 2 out]
        n254 = property on="Rev/Fwd" class="Clust (strict)"("Visible"=w406) -> ()  [unwired: 2 in, 2 out]
        n255 = property on="Test Ring" class="Ring (strict)"("Visible"=w406) -> ()  [unwired: 2 in, 2 out]
      }
      event "Select Auto": Mouse Enter {
        # "Populate the combo box with the list of autonomous options"
        n256 = event-data() -> ()  [unwired: 1 in, 1 out]
        n257 = call <vilib>:"NT Read String Array.vi"("Name"="Auto List") -> ("String Array"=w413:string[])  [unwired: 9 in, 1 out]
        n258 = property on="Select Auto" class="CmbBox"("Strings[]"=w413) -> ()  [unwired: 2 in, 2 out]
      }
      event "Select Auto": Value Change {
        # "User modified the Auto Selection. Write to NT variable so robot knows."
        n259 = event-data() -> ("NewVal"=w416:string)  [unwired: 1 in]
        n260 = call <vilib>:"NT Write String.vi"("String"=w416, "Name"="Auto Selector") -> ()  [unwired: 9 in, 1 out]
      }
      event "Command Selection": Value Change {
        # "Get the params and show in table"
        n261 = event-data() -> ("NewVal"=w422:i32)  [unwired: 1 in]
        n262 = property on="Command Selection" class="MCListbox (strict)"() -> ("ItemNames"=w420:string[][])  [unwired: 2 in, 2 out]
        n263 = call <vilib>:"WPI_DashboardUpdate Command Params.vi"("NewVal"=w422, "Commands"=w420, "Param Tbl"=w421) -> ()  [unwired: 8 in, 1 out]
      }
      event "Execute Command": Value Change {
        # "Started one, Unique ID holds\nresponse"
        n264 = event-data() -> ()  [unwired: 1 in, 1 out]
        n265 = property on="Command Selection" class="MCListbox (strict)"() -> ("ItemNames"=w433:string[][])  [unwired: 2 in, 2 out]
        n266 = Index Array(array=w433, index (row)="Command Selection", index (col)=0) -> (element=w431:string)
        n267 = call <vilib>:"Invoke Commands.vi"("Command Params"="Command Params", "Function Name"=w431) -> ("Params"=w427:u8, "Started"=w426:bool)  [unwired: 7 in, 1 out]
        n268 = Array Subset(array="Command Params", length (row)=w427) -> (w428:string[][])  [unwired: 3 in]
        n269 = Select(t="Executing" ("Cmd Status"), s=w426, f="" ("Cmd Status")) -> (s? t:f=→"Cmd Status":string)
      }
      event "Command Selection": Double Click {
        n270 = event-data() -> ("Row"=w441:i32)  [unwired: 1 in]
        n271 = property on="Command Selection" class="MCListbox (strict)"() -> ("ItemNames"=w444:string[][])  [unwired: 2 in, 2 out]
        n272 = local read "Command Params"() -> (w440:string[][])
        n273 = Index Array(array=w444, index (row)=w441, index (col)=0) -> (element=w442:string)
        n274 = call <vilib>:"Invoke Commands.vi"("Command Params"=w440, "Function Name"=w442) -> ("Params"=w439:u8, "Started"=w434:bool)  [unwired: 7 in, 1 out]
        n275 = Array Subset(array=w440, length (row)=w439) -> (w438:string[][])  [unwired: 3 in]
        n276 = Select(t="Executing" ("Cmd Status"), s=w434, f="" ("Cmd Status")) -> (s? t:f=w435:string)
        n277 = local write "Cmd Status"(w435) -> ()
      }
      event "CheckList": Double Click {
        # "Shift clears all"
        # "Update symbols on the listbox"
        n278 = event-data() -> ("PlatMods.Shift"=w446:bool, "Row"=w448:i32)  [unwired: 1 in]
        n279 = case shown="True" w446 {
          tunnel: w448 -> [w452 _]
          tunnel: 1 -> [w451 _]
          frame False {
            n280 = property on="CheckList" class="LstBox (strict)"() -> ("Item Symbols"=w450:i32[])  [unwired: 2 in, 2 out]
            n281 = Replace Array Subset(array=w450, new element=w451, index=w452) -> (w449:i32[])
            n282 = property on="CheckList" class="LstBox (strict)"("Item Symbols"=w449) -> ()  [unwired: 2 in, 2 out]
          }
          frame True {
            w453 = 0 ("Top Row")
            n283 = property on="CheckList" class="LstBox (strict)"() -> ("Number of Rows"=w455:u32)  [unwired: 2 in, 2 out]
            n284 = Initialize Array(0, w455) -> (w454:i32[])
            n285 = property on="CheckList" class="LstBox (strict)"("Top Row"=w453, "Value"=w453, "Item Symbols"=w454) -> ()  [unwired: 2 in, 2 out]
          }
        }
      }
      event "CheckList": Key Down {
        # "Update symbols on the listbox\nLeft and right keys check and uncheck"
        n286 = event-data() -> ("VKey"=w459:T21)  [unwired: 1 in]
        n287 = case shown="\"Left\", \"Right\"" w459 {
          selector: w459 -> [w464 _]
          tunnel: eventvkey."Left" ("VKey") -> [w462 _]
          frame "Left", "Right" {
            n288 = Equal?(x=w462, y=w464) -> (x = y?=w463:bool)
            n289 = Select(t=0, s=w463, f=1) -> (s? t:f=w465:i32)
            n290 = property on="CheckList" class="LstBox (strict)"() -> ("Item Symbols"=w468:i32[])  [unwired: 2 in, 2 out]
            n291 = Replace Array Subset(array=w468, new element=w465, index="CheckList") -> (w467:i32[])
            n292 = property on="CheckList" class="LstBox (strict)"("Item Symbols"=w467) -> ()  [unwired: 2 in, 2 out]
          }
          frame Default {
          }
        }
      }
      event "Motor.Enable": Value Change {
        # "When the test mode otor enable helper is set, update that\ntree row item's value"
        n293 = event-data() -> ("NewVal"=w474:bool)  [unwired: 1 in]
        n294 = Unbundle("Motor") -> ("Value"=w473:dbl)  [unwired: 1 out]
        n295 = Select(t=w473, s=w474, f=0.0) -> (s? t:f=w471:dbl)
        n296 = call <vilib>:"NT Write Number.vi"("Numeric"=w471, "Name"=w470) -> ()  [unwired: 9 in, 1 out]
      }
      event "Test Slider": Value Change {
        # "When the test mode slider helper is set, update that\ntree row item's value"
        n297 = event-data() -> ("NewVal"=w477:dbl)  [unwired: 1 in]
        n298 = call <vilib>:"NT Write Number.vi"("Numeric"=w477, "Name"=w478) -> ()  [unwired: 9 in, 1 out]
      }
      event "On/Off": Value Change {
        # "When the test mode on/off helper value is set, update that\ntree row item's value"
        n299 = event-data() -> ("NewVal"=w482:bool)  [unwired: 1 in]
        n300 = Boolean To (0,1)(Boolean=w482) -> (0, 1=w481:i16)
        n301 = call <vilib>:"NT Write Number.vi"("Numeric"=w481, "Name"=w480) -> ()  [unwired: 9 in, 1 out]
      }
      event "Rev/Fwd": Value Change {
        # "When the test mode helper value for relays is set, update that\ntree row item's value"
        n302 = event-data() -> ("NewVal.Forward"=w490:bool, "NewVal.Reverse"=w489:bool)  [unwired: 1 in]
        n303 = Boolean To (0,1)(Boolean=w490) -> (0, 1=w486:i16)
        n304 = Boolean To (0,1)(Boolean=w489) -> (0, 1=w488:i16)
        n305 = Negate(x=w488) -> (-x=w487:i16)
        n306 = Add(x=w486, y=w487) -> (x+y=w485:i16)
        n307 = call <vilib>:"NT Write Number.vi"("Numeric"=w485, "Name"=w484) -> ()  [unwired: 9 in, 1 out]
      }
      event "Test Ring": Value Change {
        # "When a test mode helper value is selected from the ring,\nset the tree item's variable to the string value"
        n308 = event-data() -> ("NewVal"=w494:u16)  [unwired: 1 in]
        n309 = property on="Test Ring" class="Ring (strict)"() -> ("Strings []"=w495:string[])  [unwired: 2 in, 2 out]
        n310 = Index Array(array=w495, index=w494) -> (element=w493:string)
        n311 = call <vilib>:"NT Write String.vi"("String"=w493, "Name"=w492) -> ()  [unwired: 9 in, 1 out]
      }
      event "Rec Mode": Value Change {
        # "Update globals for recording mode and path to read log from.\nClear when logging and let NetworkTables set path for vision to\nuse."
        n312 = event-data() -> ("NewVal"=w506:enum32{"Stop", "Record", "Playback"})  [unwired: 1 in]
        n313 = global write "WPI_DashboardLogging Global.vi" "Logging Filename"(path "") -> ()
        n314 = global write "WPI_DashboardLogging Global.vi" "Recording"(w506) -> ()
        n315 = case shown="\"Playback\"" w506 {
          tunnel: w505 -> [_ w508 w517]
          tunnel: [_ _ w516] -> w503
          tunnel: [_ _ w515] -> _
          tunnel: w501 -> [_ _ w513]
          tunnel: cluster{i32, i32} {-250, 170} -> [_ _ w512]
          tunnel: [_ _ T22 {"Image Size"=TRUE, "Image Type"=TRUE, "Pixel Value"=TRUE, "ROI Information"=TRUE, "Zoom Factor"=FALSE} ("Image Information Shown:All Elements")] -> w499
          tunnel: [_ _ TRUE ("Zoom Factor")] -> w498
          tunnel: w497 -> [_ _ w509]
          frame Default {
          }
          frame "Stop", "Record" {
            # "Place Window too"
            n316 = invoke class="VI" method="FP.Close"(reference=w508) -> (reference out=w507:refnum<vi>)  [unwired: 2 in, 2 out]
            n317 = invoke class="VI" method="Abort VI"(reference=w507) -> ()  [unwired: 2 in, 3 out]
          }
          frame "Playback" {
            n318 = call "Open Playback Panel.vi"("Offset"=w512, "DB VI Ref"=w513, "Playback in"=w517) -> ("Playback out"=w514:refnum<vi>)  [unwired: 8 in]
            n319 = register-events(w514, w509) -> (reference out=w516:refnum<event-registration>, error out=w515:errorcluster)  [unwired: 2 in]
          }
        }
        n320 = property on="Camera Image" class="ImageControl"("Image Information Shown"=w499, "Image Information Visible"=w498) -> ()  [unwired: 2 in, 2 out]
        n321 = call <vilib>:"WPI_DashboardNT Log FieldName Cache.vi"("Operation"=enum16{"Lookup/Add", "Index", "Clear"}."Clear") -> ()  [unwired: 8 in, 3 out]
      }
      event Panel Close {
        w519 = enum32{"Stop", "Record", "Playback"}."Stop" ("Rec Mode")
        # "Playback window has been closed, abort"
        n322 = event-data() -> ()  [unwired: 1 in, 4 out]
        n323 = local write "Rec Mode"(w519) -> ()
        n324 = global write "WPI_DashboardLogging Global.vi" "Recording"(w519) -> ()
      }
      event Panel Close {
        # "Abort playback window and ourself"
        n325 = event-data() -> ()  [unwired: 1 in, 4 out]
        n326 = invoke class="VI" method="FP.Close"(reference=w523) -> (reference out=w522:refnum<vi>)  [unwired: 2 in, 2 out]
        n327 = invoke class="VI" method="Abort VI"(reference=w522) -> (error out=w521:errorcluster)  [unwired: 2 in, 2 out]
        n328 = invoke class="VI" method="Abort VI"(error in=w521) -> ()  [unwired: 2 in, 3 out]
      }
      event User Event {
        n329 = event-data() -> ("IDs"=w530:cluster{"RPC field ID":u16, "Unique ID":u16}, "String"=w529:string)  [unwired: 1 in]
        n330 = Bundle("IDs"=w530, "String"=w529) -> (w528:T10)  [unwired: 1 in]
        n331 = call <vilib>:"Retrieve RPC Response.vi"("RPC Response"=w528) -> ("Output"=w526:string[][])  [unwired: 10 in]
        n332 = Build Array (concatenate)(w524, w526) -> (w525:string[][])
        n333 = local write "Command Params"(w525) -> ()
        n334 = local write "Cmd Status"("" ("Cmd Status")) -> ()
      }
      event "Tree": Double Click {
        n335 = event-data() -> ("PlatMods"=w534:T25, "Tag"=w533:string)  [unwired: 1 in]
        n336 = Unbundle(w534) -> ("Shift"=w532:bool)  [unwired: 4 out]
        n337 = Not(x=w532) -> (.not. x?=w531:bool)
        n338 = call <vilib>:"NT Update Persistence.vi"("Persistence"=w531, "Name"=w533) -> ()  [unwired: 9 in, 1 out]
      }
    }
  }
  n339 = while {
    tunnel: w64 -> [w537]
    i -> [w540]
    stop <- FALSE stop-if-true
    n340 = Wait (ms)(milliseconds to wait=u32 100) -> ()  [unwired: 1 out]
    n341 = case shown="\"Playback\"" "Rec Mode" {
      tunnel: w540 -> [_ _ w555]
      tunnel: [u32 2829099 ("Base Color") u32 11141120 ("Target Color") w544] -> w536
      frame "Stop", Default {
        # "Reset the color, extra updates don't cost much"
      }
      frame "Record" {
      }
      frame "Playback" {
        # "Playback"
        n342 = Quotient & Remainder(x=w555, y=u32 50 ("milliseconds to wait")) -> (x-y*floor(x/y)=w551:u32)  [unwired: 1 out]
        n343 = Divide(x=w551, y=u32 50 ("milliseconds to wait")) -> (x/y=w548:dbl)
        n344 = Multiply(x=6.283185307179586, y=w548) -> (x*y=w553:dbl)
        n345 = Sine(x=w553) -> (sin(x)=w552:dbl)
        n346 = Absolute Value(x=w552) -> (abs(x)=w545:dbl)
        n347 = call "Interpolate RGB Color.vi"("Proportion"=w545, "Target Color"=u32 30976, "Base Color"=u32 2829099) -> ("Result Color"=w544:u32)  [unwired: 8 in]
      }
    }
    n348 = property class="Pane"(reference=w537, "PaneColor"=w536) -> ()  [unwired: 1 in, 2 out]
  }
  n349 = local write "Dashboard Tab"(T2."Drive" ("Dashboard Tab")) -> ()
  n350 = property on="On/Off" class="Bool (strict)"("Visible"=w33) -> ()  [unwired: 2 in, 2 out]
  n351 = property on="Motor" class="Clust (strict)"("Visible"=w33) -> ()  [unwired: 2 in, 2 out]
  n352 = property on="Progress" class="Clust (strict)"("Visible"=w33) -> ()  [unwired: 2 in, 2 out]
  n353 = property on="Test Ring" class="Ring (strict)"("Visible"=w33) -> ()  [unwired: 2 in, 2 out]
  n354 = property on="Rev/Fwd" class="Clust (strict)"("Visible"=w33) -> ()  [unwired: 2 in, 2 out]
  n355 = while {
    tunnel: u16 1741 ("timeout ms (25000)") -> [w557]
    stop <- FALSE stop-if-true
    n356 = TCP Create Listener(10:w557) -> (0:w556:errorcluster, 3:w558:refnum<k5>)  [unwired: 4 in, 1 out]
    n357 = case shown="No Error" w556 {
      selector: w556 -> [w560 _]
      tunnel: w558 -> [w561 _]
      frame No Error {
        n358 = while {
          tunnel: w561 -> [w564]
          tunnel: w560 -> [w563]
          stop <- FALSE stop-if-true
          n359 = TCP Wait On Listener(8:w563, 11:w564) -> (0:w565:errorcluster, 4:w566:refnum<k5>)  [unwired: 2 in, 3 out]
          n360 = local write "TCP"(w566) -> ()
          n361 = case shown="No Error" w565 {
            frame No Error {
            }
            frame Error {
              n362 = Wait (ms)(milliseconds to wait=u32 1000) -> ()  [unwired: 1 out]
            }
          }
        }
      }
      frame Error {
        n363 = Wait (ms)(milliseconds to wait=u32 1000) -> ()  [unwired: 1 out]
      }
    }
  }
  n364 = local write "Command Selection"(u16 0 ("milliseconds to wait")) -> ()
  n365 = local write "Command Params"(string[][] [] ("Command Params")) -> ()
  n366 = global write "WPI_DashboardLogging Global.vi" "Recording"(w58) -> ()
  n367 = local write "Rec Mode"(w58) -> ()
  n368 = call <vilib>:"NT Write String.vi"("String"="Select Auto", "Name"="Auto Selector") -> ()  [unwired: 9 in, 1 out]
